vi "test_BuildAssets.vi"() -> (3 "Pass?":bool)   [LabVIEW 2019, in "Tests.SolutionBuilder.lvlib"]
uses:
  Tests.SolutionBuilder.lvlib
  SolutionBuilder/SolutionBuilder.lvclass
panel:
  out "Result paths":path[](array[path])
  out "error out":errorcluster
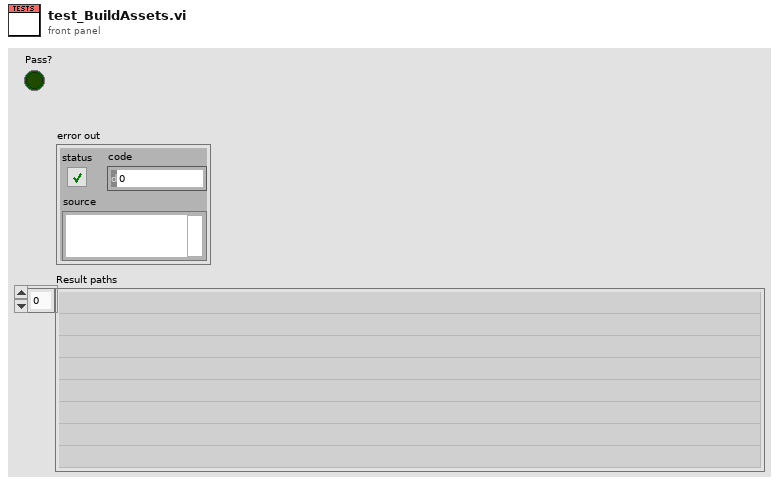
[diagram p1: front panel]
types:
  T1 = typedef "SolutionBuilder.lvlib/BuildManager.lvclass/GeneratedFile.ctl" = cluster{"Project path":path, "Build spec name":string, "Path":path}
  T2 = typedef "SolutionBuilder.lvlib/SolutionBuilder.lvclass/NamePathMap.ctl" = map{string, path}
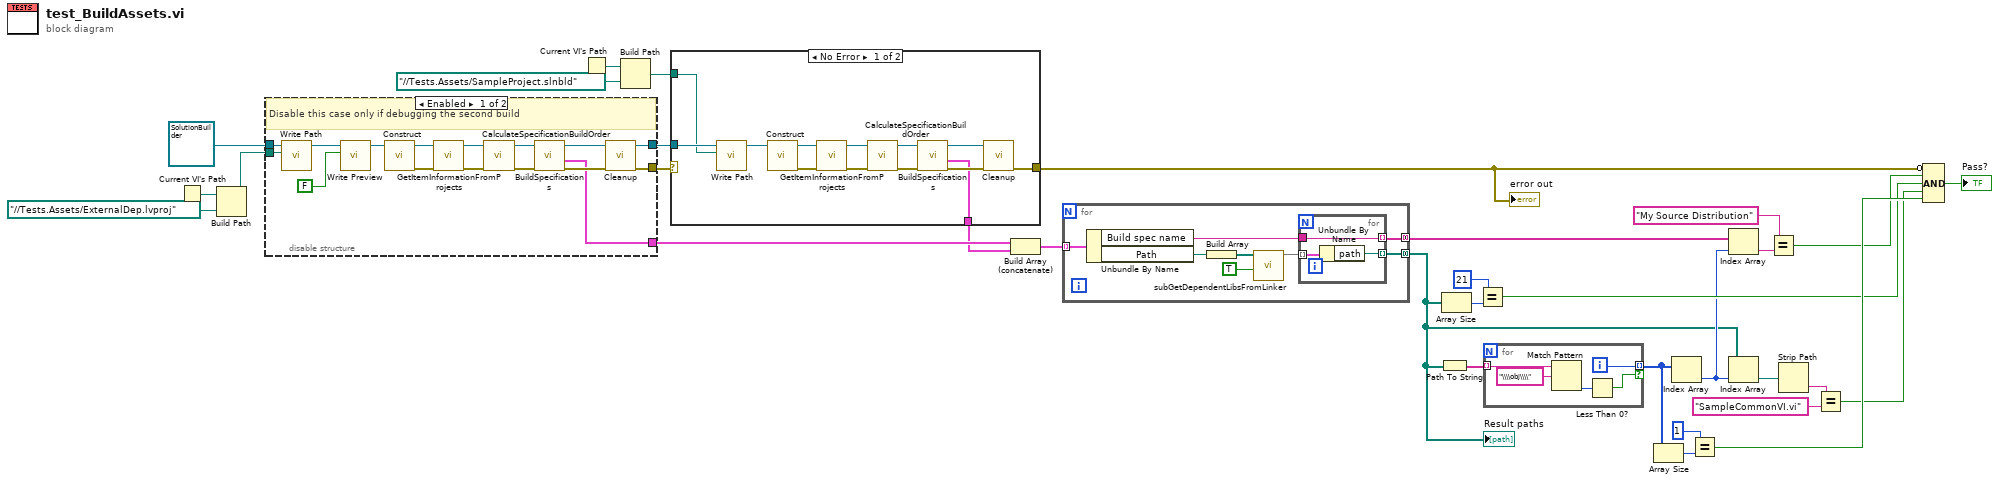
[diagram p0: block diagram]
diagram:
  n1 = Current VI's Path() -> (path=w29:path)
  n2 = Build Path(base path=w29, name or relative path=path "../../Tests.Assets/ExternalDep.lvproj" ("Path")) -> (appended path=w27:path)
  n3 = disable-structure shown="Enabled" {
    disable-tunnel: refnum<class "SolutionBuilder.lvclass"> refnum ("SolutionBuilder in") -> [w48 w49]
    disable-tunnel: w27 -> [w44 _]
    disable-tunnel: [w40 w49] -> w26
    disable-tunnel: [w38 _] -> w25
    disable-tunnel: [w37 _] -> w21
    frame Enabled {
      # "Disable this case only if debugging the second build"
      n4 = call-dynamic "Write Path.vi"("Path"=w44, "SolutionBuilder in"=w48) -> ("SolutionBuilder out"=w35:refnum<class "SolutionBuilder.lvclass">)  [unwired: 9 in]
      n5 = call-dynamic "Write Preview.vi"("Preview?"=FALSE, "SolutionBuilder in"=w35) -> ("SolutionBuilder out"=w34:refnum<class "SolutionBuilder.lvclass">)  [unwired: 9 in]
      n6 = call-dynamic "Construct.vi"("SolutionBuilder in"=w34) -> ("error out"=w43:errorcluster, "SolutionBuilder out"=w47:refnum<class "SolutionBuilder.lvclass">)  [unwired: 9 in]
      n7 = call-dynamic "GetItemInformationFromProjects.vi"("error in (no error)"=w43, "SolutionBuilder in"=w47) -> ("error out"=w42:errorcluster, "SolutionBuilder out"=w46:refnum<class "SolutionBuilder.lvclass">)  [unwired: 8 in]
      n8 = call-dynamic "CalculateSpecificationBuildOrder.vi"("error in (no error)"=w42, "SolutionBuilder in"=w46) -> ("error out"=w41:errorcluster, "SolutionBuilder out"=w45:refnum<class "SolutionBuilder.lvclass">)  [unwired: 8 in]
      n9 = call-dynamic "BuildSpecifications.vi"("error in (no error)"=w41, "SolutionBuilder in"=w45) -> ("error out"=w39:errorcluster, "Generated files"=w37:T1[], "SolutionBuilder out"=w36:refnum<class "SolutionBuilder.lvclass">)  [unwired: 7 in]
      n10 = call-dynamic "Cleanup.vi"("error in (no error)"=w39, "SolutionBuilder in"=w36) -> ("error out"=w38:errorcluster, "SolutionBuilder out"=w40:refnum<class "SolutionBuilder.lvclass">)  [unwired: 8 in]
    }
    frame Disabled {
    }
  }
  n11 = Current VI's Path() -> (path=w24:path)
  n12 = Build Path(base path=w24, name or relative path=path "../../Tests.Assets/SampleProject.slnbld" ("Path")) -> (appended path=w22:path)
  n13 = case shown="No Error" w25 {
    selector: w25 -> [_ w63]
    tunnel: w26 -> [w55 _]
    tunnel: [w53 w63] -> w32
    tunnel: w22 -> [w52 _]
    tunnel: [w51 _] -> w20
    frame No Error {
      n14 = call-dynamic "Write Path.vi"("Path"=w52, "SolutionBuilder in"=w55) -> ("SolutionBuilder out"=w56:refnum<class "SolutionBuilder.lvclass">)  [unwired: 9 in]
      n15 = call-dynamic "Construct.vi"("SolutionBuilder in"=w56) -> ("error out"=w60:errorcluster, "SolutionBuilder out"=w57:refnum<class "SolutionBuilder.lvclass">)  [unwired: 9 in]
      n16 = call-dynamic "GetItemInformationFromProjects.vi"("error in (no error)"=w60, "SolutionBuilder in"=w57) -> ("error out"=w61:errorcluster, "SolutionBuilder out"=w58:refnum<class "SolutionBuilder.lvclass">)  [unwired: 8 in]
      n17 = call-dynamic "CalculateSpecificationBuildOrder.vi"("error in (no error)"=w61, "SolutionBuilder in"=w58) -> ("error out"=w62:errorcluster, "SolutionBuilder out"=w59:refnum<class "SolutionBuilder.lvclass">)  [unwired: 8 in]
      n18 = call-dynamic "BuildSpecifications.vi"("error in (no error)"=w62, "SolutionBuilder in"=w59) -> ("error out"=w54:errorcluster, "Generated files"=w51:T1[], "SolutionBuilder out"=w50:refnum<class "SolutionBuilder.lvclass">)  [unwired: 7 in]
      n19 = call-dynamic "Cleanup.vi"("error in (no error)"=w54, "SolutionBuilder in"=w50) -> ("error out"=w53:errorcluster)  [unwired: 8 in, 1 out]
    }
    frame Error {
    }
  }
  "error out" <- w32
  n20 = Build Array (concatenate)(w21, w20) -> (w4:T1[])
  n21 = for {
    tunnel: w4 -> [w71] mode=indexing
    tunnel: [w65] -> w3 mode=concatenating
    tunnel: [w64] -> w1 mode=concatenating
    n22 = Unbundle By Name(w71) -> ("Build spec name"=w66:string, "Path"=w70:path)
    n23 = Build Array(w70) -> (w67:path[])
    n24 = call "subGetDependentLibsFromLinker.vi"("All?"=TRUE, "Paths"=w67) -> ("Dependency libs"=w69:T2)  [unwired: 9 in]
    n25 = for {
      tunnel: [w73] -> w64 mode=indexing
      tunnel: w69 -> [w74] mode=indexing
      tunnel: [w72] -> w65 mode=indexing
      tunnel: w66 -> [w72]
      n26 = Unbundle By Name(w74) -> ("path"=w73:path)
    }
  }
  "Result paths" <- w1
  n27 = Path To String(path=w1) -> (string=w19:string[])
  n28 = Array Size(array=w1) -> (size(s)=w18:i32)
  n29 = Equal?(x=21, y=w18) -> (x = y?=w8:bool)
  n30 = for {
    tunnel: w19 -> [w79] mode=indexing
    tunnel: [w75] -> w14 mode=indexing if=w76
    i -> [w75]
    n31 = Match Pattern(string=w79, regular expression="\\\\obj\\\\") -> (offset past match=w77:i32)  [unwired: 1 in, 3 out]
    n32 = Less Than 0?(x=w77) -> (x < 0?=w76:bool)
  }
  n33 = Array Size(array=w14) -> (size(s)=w15:i32)
  n34 = Index Array(array=w14) -> (element=w7:i32)  [unwired: 1 in]
  n35 = Equal?(x=1, y=w15) -> (x = y?=w10:bool)
  n36 = Index Array(array=w3, index=w7) -> (element=w2:string)
  n37 = Index Array(array=w1, index=w7) -> (element=w13:path)
  n38 = Equal?(x="My Source Distribution" ("regular expression"), y=w2) -> (x = y?=w5:bool)
  n39 = Strip Path(path=w13) -> (name=w12:string)  [unwired: 1 out]
  n40 = Equal?(x=w12, y="SampleCommonVI.vi" ("regular expression")) -> (x = y?=w9:bool)
  n41 = Compound Arithmetic op=AND(invert w32, w5, w8, w9, w10) -> (→"Pass?":bool)
